vi "sv_Filter Even-Angle Signal for All Harmonics.vi"(0 "even-angle signals":cluster{"r0":dbl, "dr":dbl, "Y":dbl[]}[](array[cluster]), 2 "reset?":bool, 7 "even-angle position info":T1, 9 "harmonic range":cluster{"start":dbl, "stop":dbl}={"start"=-1.0, "stop"=-1.0} {"stop" format="%.2f"; "start" format="%.2f"}, 11 "error in (no error)":errorcluster, 13 "zero delay? (F)":bool) -> (4 "even-angle signals out":cluster{"r0":dbl, "dr":dbl, "Y":dbl[]}[](array[cluster]), 8 "even-angle position info out":T1, 15 "error out":errorcluster)   [LabVIEW 2017, in "SoundVib_ContSweptSine.lvlib"]
uses:
  <vilib>/addons/Sound and Vibration/svt_Continuous Swept Sine/SoundVib_ContSweptSine.lvlib
  <vilib>/addons/Sound and Vibration/Order Analysis/Misc/OAT Position Info.ctl
  <vilib>/Analysis/3filter.llb/FIR Filter with I.C. (DBL).vi
  <vilib>/Analysis/NI_AALBase.lvlib
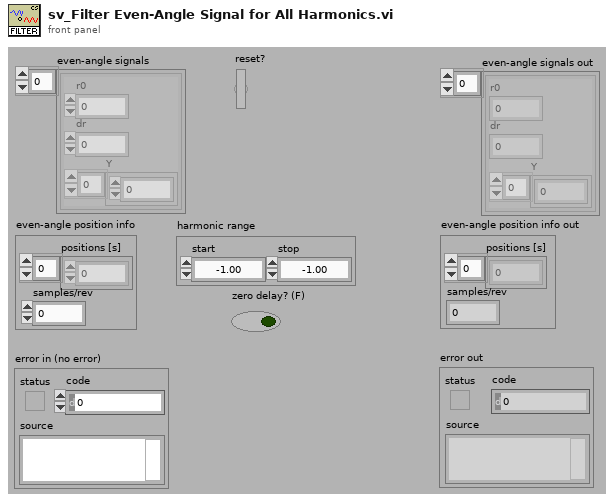
[diagram p1: front panel]
types:
  T1 = typedef "OAT Position Info.ctl" = cluster{"positions [s]":dbl[], "samples/rev":dbl}
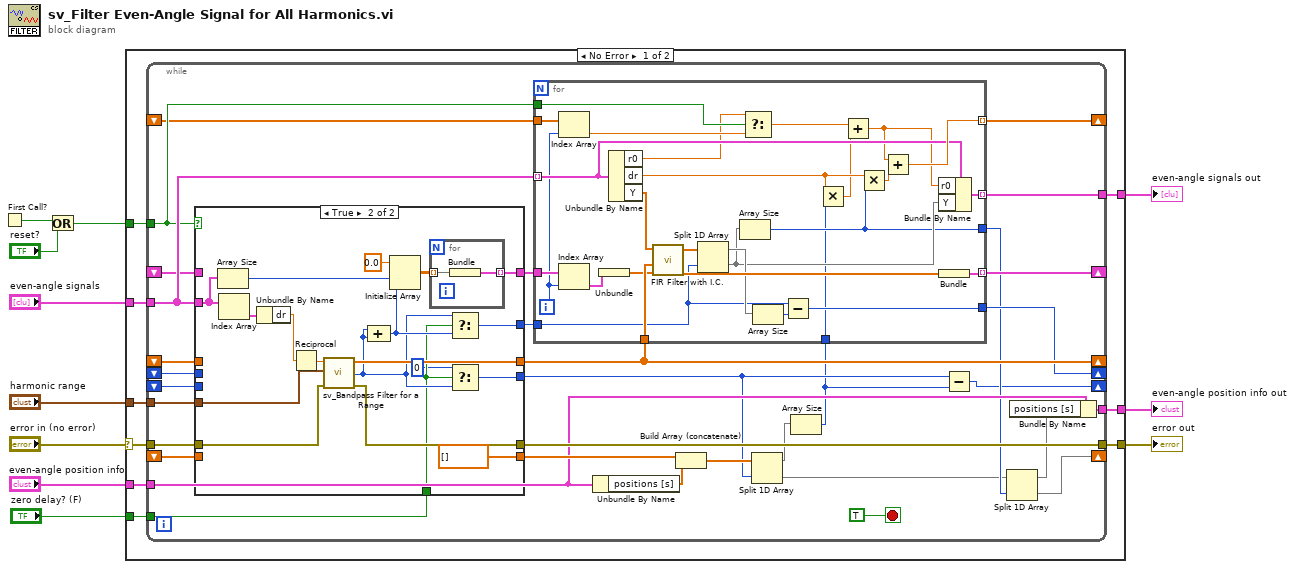
[diagram p0: block diagram]
diagram:
  n1 = First Call?() -> (First Call?: T/F=w11:bool)
  n2 = Or(x=w11, y="reset?") -> (x .or. y?=w9:bool)
  n3 = case shown="No Error" "error in (no error)" {
    selector: "error in (no error)" -> [w16 w111]
    tunnel: w9 -> [w20 _]
    tunnel: "even-angle signals" -> [w19 w110]
    tunnel: "harmonic range" -> [w18 _]
    tunnel: [w17 w110] -> w7
    tunnel: [w15 w111] -> w5
    tunnel: "even-angle position info" -> [w14 w109]
    tunnel: [w13 w109] -> w3
    tunnel: "zero delay? (F)" -> [w12 _]
    frame No Error {
      n4 = while {
        tunnel: w20 -> [w45]
        tunnel: w19 -> [w48]
        tunnel: w18 -> [w52]
        shift-right: [w47] -> _
        shift-left: _ -> [w51]
        shift-right: [w46] -> _
        shift-left: _ -> [w41]
        shift-right: [w49] -> _
        shift-left: _ -> [w40]
        shift-right: [w44] -> _
        shift-left: _ -> [w43]
        tunnel: [w42] -> w17
        tunnel: w16 -> [w39]
        tunnel: [w38] -> w15
        tunnel: w14 -> [w31]
        shift-right: [w36] -> _
        shift-left: _ -> [w35]
        tunnel: [w30] -> w13
        tunnel: w12 -> [w24]
        shift-right: [w26] -> _
        shift-left: _ -> [w25]
        stop <- TRUE stop-if-true
        n5 = case shown="True" w45 {
          tunnel: w48 -> [_ w101]
          tunnel: w52 -> [_ w94]
          tunnel: [w87 w103] -> w47
          tunnel: w51 -> [w87 _]
          tunnel: [w86 w98] -> w50
          tunnel: w41 -> [w82 _]
          tunnel: w40 -> [w86 _]
          tunnel: w39 -> [w85 w97]
          tunnel: [w85 w96] -> w38
          tunnel: w35 -> [w84 _]
          tunnel: [w84 dbl[] []] -> w33
          tunnel: [w83 w88] -> w22
          tunnel: w25 -> [w83 _]
          tunnel: w24 -> [_ w90]
          tunnel: [w82 w92] -> w23
          frame False {
          }
          frame True {
            n6 = Array Size(array=w101) -> (size(s)=w100:i32)
            n7 = Index Array(array=w101) -> (element=w106:cluster{"r0":dbl, "dr":dbl, "Y":dbl[]})  [unwired: 1 in]
            n8 = Unbundle By Name(w106) -> ("dr"=w104:dbl)
            n9 = Reciprocal(x=w104) -> (1/x=w105:dbl)
            n10 = call <vilib>:"sv_Bandpass Filter for a Range.vi"("error in (no error)"=w97, "harmonic range"=w94, "fs"=w105) -> ("error out"=w96:errorcluster, "delay [samples]"=w91:i32, "FIR filter"=w103:dbl[])  [unwired: 6 in]
            n11 = Compound Arithmetic op=ADD(w91, w91) -> (w93:i32)
            n12 = Initialize Array(0.0 ("element"), w100, w93) -> (w99:dbl[][])
            n13 = for {
              tunnel: w99 -> [w108] mode=indexing
              tunnel: [w107] -> w98 mode=indexing
              n14 = Bundle(w108) -> (w107:cluster{dbl[]})  [unwired: 1 in]
            }
            n15 = Select(t=w91, s=w90, f=w93) -> (s? t:f=w92:i32)
            n16 = Select(t=0, s=w90, f=w91) -> (s? t:f=w88:i32)
          }
        }
        n17 = Unbundle By Name(w31) -> ("positions [s]"=w37:dbl[])
        n18 = Build Array (concatenate)(w33, w37) -> (w34:dbl[])
        n19 = Split 1D Array(array=w34, index=w22) -> (first subarray=w27:dbl[], second subarray=w28:dbl[])
        n20 = Array Size(array=w27) -> (size(s)=w21:i32)
        n21 = for {
          tunnel: w50 -> [w81]
          tunnel: [w65] -> w49 mode=indexing
          tunnel: w48 -> [w71] mode=indexing
          tunnel: w47 -> [w78]
          tunnel: [w75] -> w46
          tunnel: w45 -> [w69]
          tunnel: [w72] -> w44 mode=indexing
          tunnel: w43 -> [w68]
          tunnel: [w66] -> w42 mode=indexing
          tunnel: [w60] -> w29
          tunnel: w23 -> [w59]
          tunnel: w21 -> [w58]
          i -> [w61]
          n22 = Index Array(array=w68, index=w61) -> (element=w63:dbl)
          n23 = Index Array(array=w81, index=w61) -> (element=w62:cluster{"Final X Conditions":dbl[]})
          n24 = Unbundle(w62) -> ("Final X Conditions"=w64:dbl[])
          n25 = Unbundle By Name(w71) -> ("r0"=w56:dbl, "dr"=w57:dbl, "Y"=w79:dbl[])
          n26 = call-poly <vilib>:"FIR Filter with I.C..vi"("Initial X Conditions"=w64, "FIR Coefficients"=w78, "X"=w79) -> ("Final X Conditions"=w80:dbl[], "Filtered X"=w77:dbl[])  [unwired: 5 in, 1 out]
          n27 = Split 1D Array(array=w77, index=w59) -> (first subarray=w74:dbl[], second subarray=w70:dbl[])
          n28 = Array Size(array=w70) -> (size(s)=w60:i32)
          n29 = Select(t=w56, s=w69, f=w63) -> (s? t:f=w67:dbl)
          n30 = Array Size(array=w74) -> (size(s)=w76:i32)
          n31 = Subtract(x=w59, y=w76) -> (x-y=w75:i32)
          n32 = Multiply(x=w57, y=w58) -> (x*y=w55:dbl)
          n33 = Add(x=w67, y=w55) -> (x+y=w54:dbl)
          n34 = Multiply(x=w57, y=w60) -> (x*y=w73:dbl)
          n35 = Add(x=w54, y=w73) -> (x+y=w72:dbl)
          n36 = Bundle By Name(cluster=w71, "r0"=w54, "Y"=w70) -> (w66:cluster{"r0":dbl, "dr":dbl, "Y":dbl[]})
          n37 = Bundle("Final X Conditions"=w80) -> (w65:cluster{"Final X Conditions":dbl[]})  [unwired: 1 in]
        }
        n38 = Subtract(x=w22, y=w21) -> (x-y=w26:i32)
        n39 = Split 1D Array(array=w28, index=w29) -> (first subarray=w32:dbl[], second subarray=w36:dbl[])
        n40 = Bundle By Name(cluster=w31, "positions [s]"=w32) -> (w30:T1)
      }
    }
    frame Error {
    }
  }
  "even-angle signals out" <- w7
  "error out" <- w5
  "even-angle position info out" <- w3
